vi "PSVCH_Get Data.vi"(8 "Error In (no error)":errorcluster, 10 "Time Out(10)":i32=10, 11 "CHTag":string) -> (0 "Error Out":errorcluster, 2 "timed out?":bool, 3 "Data":waveform(dbl)[](array[waveform]))   [LabVIEW 2016]
panel:
  # "Data Out"
  # "Data In"
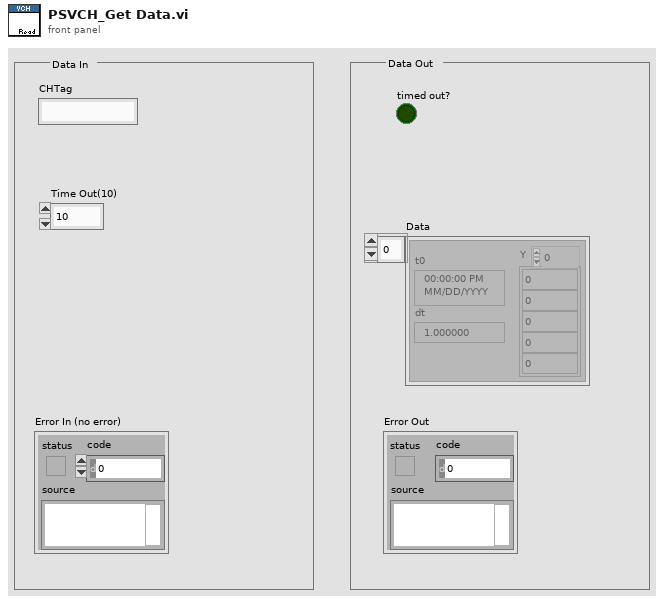
[diagram p1: front panel]
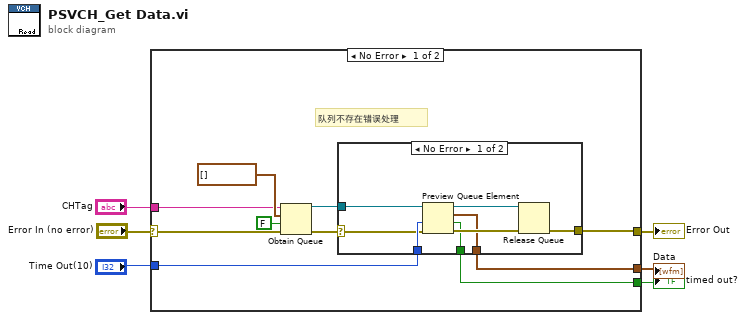
[diagram p0: block diagram]
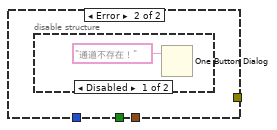
[diagram p2: hidden frame]
diagram:
  n1 = case shown="No Error" "Error In (no error)" {
    selector: "Error In (no error)" -> [w13 w26]
    tunnel: [w14 w26] -> w5
    tunnel: "CHTag" -> [w11 _]
    tunnel: "Time Out(10)" -> [w10 _]
    tunnel: [w9 _] -> w2
    tunnel: [w8 _] -> w1
    frame No Error {
      # "队列不存在错误处理"
      n2 = Obtain Queue(name (unnamed)=w11, element data type=waveform(dbl)[] [] ("Out"), create if not found? (T)=FALSE ("如未找到是否创建？(T)"), error in (no error)=w13) -> (queue out=w16:refnum<queue>, error out=w7:errorcluster)  [unwired: 1 in, 1 out]
      n3 = case shown="No Error" w7 {
        selector: w7 -> [w17 _]
        tunnel: w16 -> [w22 _]
        tunnel: [w21 _] -> w14
        tunnel: w10 -> [w20 _]
        tunnel: [w19 _] -> w9
        tunnel: [w18 _] -> w8
        frame No Error {
          n4 = Preview Queue Element(queue=w22, timeout in ms (-1)=w20, error in (no error)=w17) -> (queue out=w23:refnum<queue>, element=w19:waveform(dbl)[], timed out?=w18:bool, error out=w24:errorcluster)
          n5 = Release Queue(queue=w23, error in (no error)=w24) -> (error out=w21:errorcluster)  [unwired: 1 in, 2 out]
        }
        frame Error {
          n6 = disable-structure shown="Disabled" {
            frame Disabled {
              n7 = One Button Dialog(message="通道不存在！") -> ()  [unwired: 1 in, 1 out]
            }
            frame Enabled {
            }
          }
        }
      }
    }
    frame Error {
    }
  }
  "Error Out" <- w5
  "Data" <- w2
  "timed out?" <- w1
